vi "Get Resize Offsets 1d.vi"(8 "error in (no error)":errorcluster, 10 "TBL1D Refnum":refnum<vi>, 11 "Pane in":refnum<vi>) -> (0 "error out":errorcluster, 2 "Width Offset":u32, 3 "Height Offset":u32)   [LabVIEW 2011]
uses:
  Tables/XCPCCP TBL1D.xctl
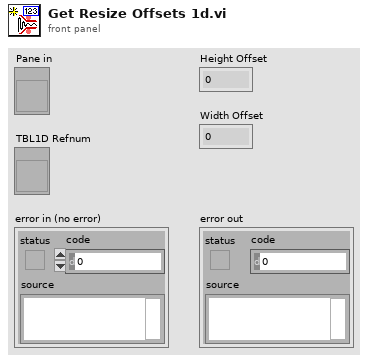
[diagram p1: front panel]
types:
  T1 = typedef "LVBoundsTypeDef.ctl" = cluster{"Width":u32, "Height":u32}
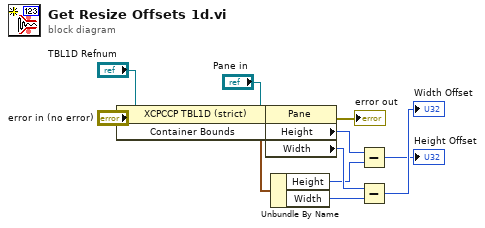
[diagram p0: block diagram]
diagram:
  n1 = property on="Property Node" class="XCPCCP TBL1D (strict)"(reference="TBL1D Refnum", error in="error in (no error)") -> (error out=w7:errorcluster, "Container Bounds"=w5:T1)  [unwired: 1 out]
  n2 = property on="Property Node" class="Pane"(reference="Pane in", error in=w7) -> (error out=→"error out":errorcluster, "Height"=w4:u32, "Width"=w11:u32)  [unwired: 1 out]
  n3 = Unbundle By Name(w5) -> ("Height"=w6:u32, "Width"=w9:u32)
  n4 = Subtract(x=w4, y=w6) -> (x-y=→"Height Offset":u32)
  n5 = Subtract(x=w11, y=w9) -> (x-y=→"Width Offset":u32)
